vi "Store Visibility.vi"(8 "error in (no error)":errorcluster, 10 "Visibility Data":T1, 11 "GUI Manager Module in":refnum<class "GUI Manager Module.lvclass">) -> (0 "error out":errorcluster, 3 "GUI Manager Module out":refnum<class "GUI Manager Module.lvclass">)   [LabVIEW 2020, in "VolatusGUI.lvlib" / "GUI Manager Module.lvclass"]
uses:
  GUI Manager Module.lvclass
  Visibility Data.ctl
  GUI Manager Module.lvclass/GUI Manager Module.ctl
  lv-vecto/Vecto/Vecto.lvlib
  lv-userprefs/User Prefs/Pref Group/Pref Group.lvclass
  VolatusGUI.lvlib
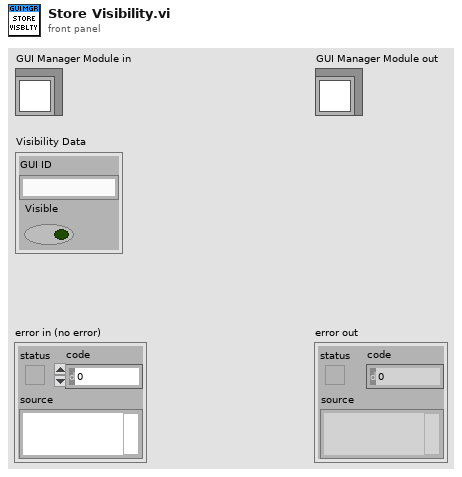
[diagram p1: front panel]
types:
  T1 = typedef "VolatusGUI.lvlib/Visibility Data.ctl" = cluster{"GUI ID":string, "Visible":bool}
  T2 = typedef "VolatusGUI.lvlib/GUI Registration.ctl" = cluster{"ID":string, "GUI Helper":refnum<class "MessageQ.lvclass">, "Module":refnum<class "MessageQ.lvclass">, "Info":T3, "Open":bool}
  T3 = typedef "VolatusGUI.lvlib/GUI Info.ctl" = cluster{"Color":u32, "Name":string}
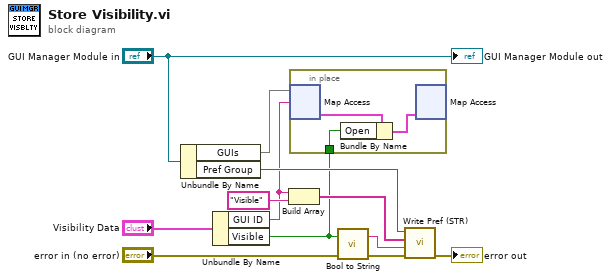
[diagram p0: block diagram]
diagram:
  n1 = Unbundle By Name("GUI Manager Module in") -> ("GUIs"=w3:map{string, T2}, "Pref Group"=w8:refnum<class "Pref Group.lvclass">)
  n2 = Unbundle By Name("Visibility Data") -> ("GUI ID"=w2:string, "Visible"=w1:bool)
  n3 = Build Array(w2, "Visible" ("element")) -> (w4:string[])
  n4 = in-place {
    in-place-border: w1 -> [w13]
    n5 = in-place-map #1(w3, w2) -> (w14:T2)  [unwired: 1 in, 1 out]
    n6 = Bundle By Name(cluster=w14, "Open"=w13) -> (w12:T2)
    n7 = in-place-map #1(w12) -> ()  [unwired: 1 in, 3 out]
  }
  n8 = call "Bool to String.vi"("Bool"=w1) -> ("String"=w5:string)  [unwired: 2 in]
  n9 = call "Write Pref (STR).vi"("error in (no error)"="error in (no error)", "Value"=w5, "Pref Hierarchy"=w4, "Pref Group in"=w8) -> ("error out"=→"error out":errorcluster)  [unwired: 6 in, 1 out]
  "GUI Manager Module out" <- "GUI Manager Module in"
